vi "Read TxPkt Decimation.vi"(8 "error in (no error)":errorcluster, 11 "Node Ptr":T1 format="%.0x") -> (0 "error out":errorcluster, 2 "Decimation":u16, 3 "Node Ptr out":T1 format="%.0x")   [LabVIEW 2019, in "UDP-Custom-Device System Explorer.lvlib" / "Tx Packet Accessors.lvlib"]
uses:
  Tx Packet Accessors.lvlib
  <vilib>/NI VeriStand/Custom Device API/Custom Device Item Ref.ctl
  Shared/Constants.vi
  <vilib>/NI VeriStand/Custom Device API/Get Item Property (U16).vi
  <vilib>/NI VeriStand/Custom Device API/Custom Device API.lvlib
  Shared/UDP-Custom-Device Shared.lvlib
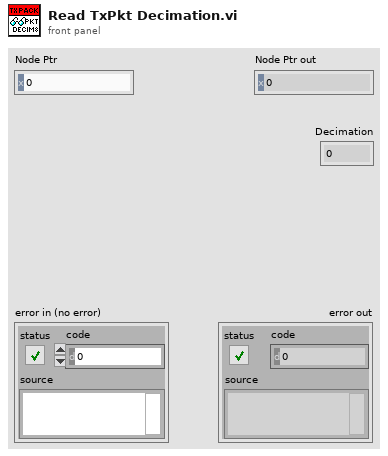
[diagram p1: front panel]
types:
  T1 = typedef "Custom Device API.lvlib/Custom Device Item Ref.ctl" = u64
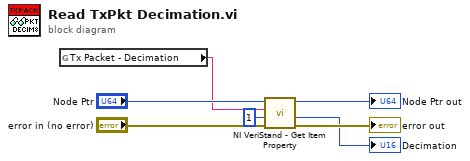
[diagram p0: block diagram]
diagram:
  n1 = global read "Constants.vi" "Tx Packet - Decimation"() -> (w3:string)
  n2 = call-poly <vilib>:"NI VeriStand - Get Item Property.vi"("error in (no error)"="error in (no error)", "Default Value"=u16 1, "Property Name"=w3, "Item Ref in"="Node Ptr") -> ("error out"=→"error out":errorcluster, "Value"=→"Decimation":u16, "Item Ref out"=→"Node Ptr out":T1)  [unwired: 4 in, 1 out]
